vi "RecursiveSequence.vi"() -> ()   [LabVIEW 2014]
panel:
  in  "N terms":i32=30
  in  "y0 through y2":dbl[](array[numeric])=[0.0, 1.0, 2.0]
  out "Y":dbl[](array[numeric])
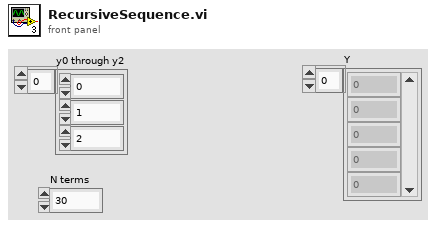
[diagram p1: front panel]
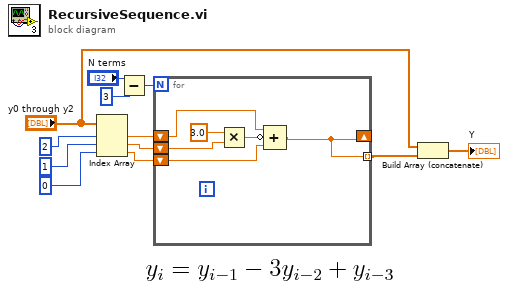
[diagram p0: block diagram]
diagram:
  n1 = Index Array(array="y0 through y2", index #1=2 ("index"), index #2=1 ("index"), index #3=0 ("index")) -> (element #1=w7:dbl, element #2=w6:dbl, element #3=w1:dbl)
  n2 = Subtract(x="N terms", y=3) -> (x-y=w8:i32)
  n3 = for {
    N: w8 -> [_]
    shift-right: [w13] -> _
    shift-left: w7 -> [w15]
    shift-left: w6 -> [w17]
    tunnel: [w13] -> w5 mode=indexing
    shift-left: w1 -> [w14]
    n4 = Multiply(x=3.0, y=w17) -> (x*y=w16:dbl)
    n5 = Compound Arithmetic op=ADD(w15, invert w16, w14) -> (w13:dbl)
  }
  n6 = Build Array (concatenate)("y0 through y2", w5) -> (→"Y":dbl[])
